vi "config channel.vi"(7 "sample mode":i32(ring)=10178 items=["Finite Samples"=10178, "Continuous Samples"=10123, "Hardware Timed Single Point"=12522], 8 "error in":errorcluster, 11 "DAQ Config":T1) -> (0 "error out":errorcluster, 3 "DAQ Config out":T1)   [LabVIEW 2017, in "Acquisition.lvlib"]
uses:
  Acquisition.lvlib
  Control/Config chanel.ctl
  <vilib>/DAQmx/create/channels.llb/DAQmx Create Channel (AI-Voltage-Basic).vi
  <vilib>/DAQmx/configure/timing.llb/DAQmx Timing (Sample Clock).vi
panel:
  out "Error":bool
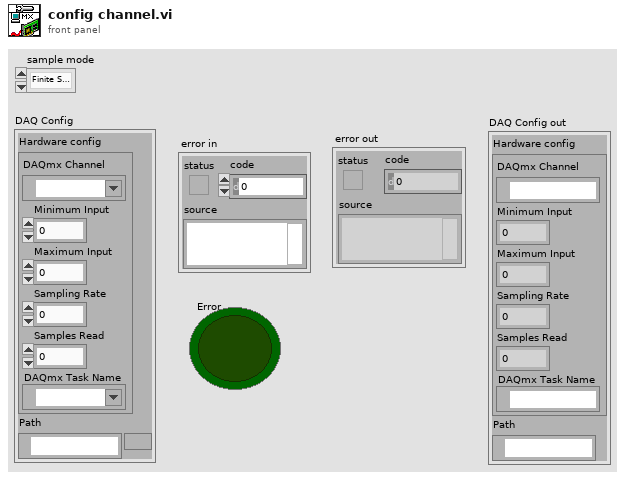
[diagram p1: front panel]
types:
  T1 = typedef "Config chanel.ctl" = cluster{"Hardware config":cluster{"DAQmx Channel":tag, "Minimum Input":dbl, "Maximum Input":dbl, "Sampling Rate":dbl, "Samples Read":dbl, "DAQmx Task Name":refnum<k21>}, "Path":path}
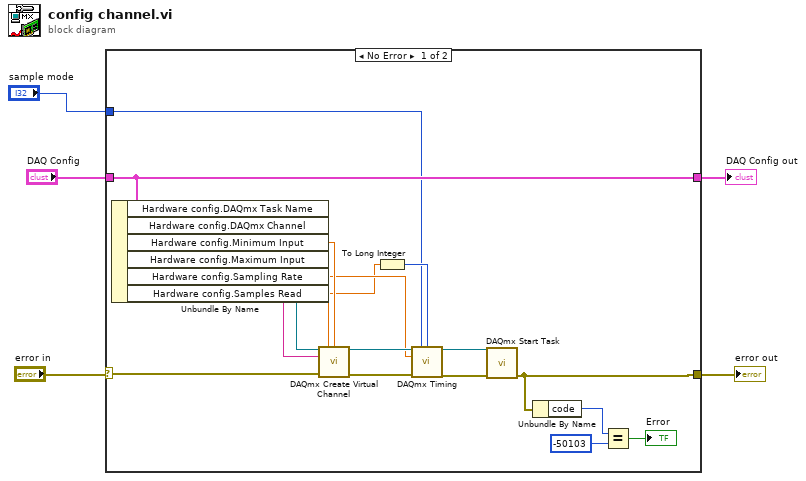
[diagram p0: block diagram]
diagram:
  n1 = case shown="No Error" "error in" {
    selector: "error in" -> [w11 w24]
    tunnel: [w8 w24] -> w5
    tunnel: [w23 w25] -> w3
    tunnel: "DAQ Config" -> [w23 w25]
    tunnel: "sample mode" -> [w6 _]
    frame No Error {
      n2 = Unbundle By Name(w23) -> ("Hardware config.DAQmx Task Name"=w22:refnum<k21>, "Hardware config.DAQmx Channel"=w21:tag, "Hardware config.Minimum Input"=w20:dbl, "Hardware config.Maximum Input"=w19:dbl, "Hardware config.Sampling Rate"=w14:dbl, "Hardware config.Samples Read"=w13:dbl)
      n3 = call-poly <vilib>:"DAQmx Create Virtual Channel.vi"("task in"=w22, "maximum value"=w19, "minimum value"=w20, "physical channels"=w21, "error in"=w11) -> ("task out"=w18:refnum<k21>, "error out"=w17:errorcluster)  [unwired: 9 in]
      n4 = To Long Integer(number=w13) -> (32bit integer=w12:i32)
      n5 = call-poly <vilib>:"DAQmx Timing.vi"("task/channels in"=w18, "sample mode"=w6, "samples per channel"=w12, "rate"=w14, "error in"=w17) -> ("task out"=w16:refnum<k21>, "error out"=w15:errorcluster)  [unwired: 9 in]
      n6 = call <vilib>:"DAQmx Start Task.vi"("task/channels in"=w16, "error in"=w15) -> ("error out"=w8:errorcluster)  [unwired: 12 in, 1 out]
      n7 = Unbundle By Name(w8) -> ("code"=w10:i32)
      n8 = Equal?(x=w10, y=-50103) -> (x = y?=→"Error":bool)
    }
    frame Error {
    }
  }
  "DAQ Config out" <- w3
  "error out" <- w5
